vi "Main.vi"() -> ()   [LabVIEW 2021]
uses:
  <vilib>/Analysis/NI_AALBase.lvlib
  <vilib>/Analysis/Matrix/NI_Matrix.lvlib
  <vilib>/Analysis/baseanly.llb/Real Inverse Matrix.vi
  <vilib>/Analysis/Matrix/Numeric/Multiply/Multiply - RM,RM.vi
  <vilib>/Analysis/NI_AALPro.lvlib
  <vilib>/gmath/NI_Gmath.lvlib
  <vilib>/Analysis/7linalg.llb/Eigenvalue and Vectors Output Option.ctl
  <vilib>/Analysis/7linalg.llb/Real Eigenvalues and Vectors.vi
  <vilib>/Analysis/baseanly.llb/Matrix Type of Inverse Matrix.ctl
  <vilib>/Analysis/Matrix/Numeric/Conversions/Array To Matrix - RA2.vi
  <vilib>/Analysis/4window.llb/Hanning Window (DBL).vi
  <vilib>/Analysis/5stat.llb/RMS (DBL).vi
  <vilib>/DAQmx/read.llb/DAQmx Read (Analog 1D DBL 1Chan NSamp).vi
  <vilib>/Analysis/Matrix/Numeric/Add/Add - RM,RM.vi
  <vilib>/Analysis/7linalg.llb/Real Cholesky Factorization.vi
  <vilib>/Analysis/2dsp.llb/Real FFT.vi
  <vilib>/Analysis/baseanly.llb/Mean (DBL).vi
  <vilib>/Analysis/7linalg.llb/Real Generalized Eigenvalues and Vectors.vi
  <vilib>/DAQmx/write.llb/DAQmx Write (Digital 1D Bool NChan 1Samp 1Line).vi
  <vilib>/gmath/statdist.llb/Normal Moments.vi
panel:
  out "Waveform Graph":dbl[](graph)
  out "1st Nat. Freq. (Hz) 4":waveform(dbl)[](graph) caption="1st Nat. Freq. (Hz)"
  out "1st Nat. Freq. (Hz) 3":waveform(dbl)(graph) caption="Est. 1st Nat. Freq. (Hz)"
  out "Std. Dev.":dbl
  in  "error in 2":errorcluster caption="error in"
  out "time_acceleration_data":dbl[](array[numeric])
  out "XY Graph 2":cluster{dbl[], dbl[]}[](graph)
  in  "MASTER":bool
  out "XY Graph":cluster{dbl[], dbl[]}[](graph)
  out "1st Nat. Freq. (Hz)":waveform(dbl)(graph) caption="measured 1st Nat. Freq. (Hz)"
  out "Estimated Pin Node":i32[](graph)
  in  "Tab Control":T1(tab)
  in  "Frequency Method":enum16{"0-Tone", "1-FFT-CPU"}(ring)=enum."1-FFT-CPU"
  in  "Width":dbl=0.0508 format="%#.6f"
  in  "Density":dbl=7900.0
  in  "Height":dbl=0.00635
  in  "Length of Beam":dbl=0.3525
  in  "Young's Modulus":dbl=209500000000.0
  in  "Torsion Spring":dbl format="%#.6f"
  in  "Initial Pin node":i32
  in  "Std. Dev.":dbl=1.0 min=0.0
  in  "Eigenvalue Method":T2(ring)=enum."2-LabVIEW Cholesky Factorization"
  out "average cycle time (ms)":dbl format="%0.2f"
  in  "FFT data length (data points)":i32=5000
  in  "Min. FFT Power Value (RMS)":dbl=0.02
  in  "Bound to 1st Frequency":bool=TRUE
  out "Low-Energy Warning":bool
  in  "accelerometer_mass":dbl=0.055
  in  "Std. Dev = Number of Particles / 3":bool=TRUE
  out "Std. Dev.  2":dbl
  in  "Number Of Particles":i32=3
  in  "FEA Nodes":i32=40
  in  "file name":i32
  out "FFT_data_length":i32=5000
  in  "Auto FFT length":bool
  out "Hz / per pin location":dbl
  out "FFT_frequency_resolution":dbl
  in  "scaling_factor_Hz_per_pin_to_frequency_resolution":dbl=0.33 format="%#_13g"
  in  "save acceleration_data":bool=TRUE
  out "1st Nat. Freq. (Hz) 2":dbl format="%#_5g"
  out "FEA Frequencies":dbl[](array[numeric])
  out "Acceleration Data":dbl[](graph) caption="All Data"
  out "Sampled Acceleration Data":dbl[](graph) caption="Sampled Data"
  in  "Real-Time plotting":bool
  out "Probability Density Function":cluster{i32[], dbl[]}(graph)
  # "Note: All Inputs are based on base SI units."
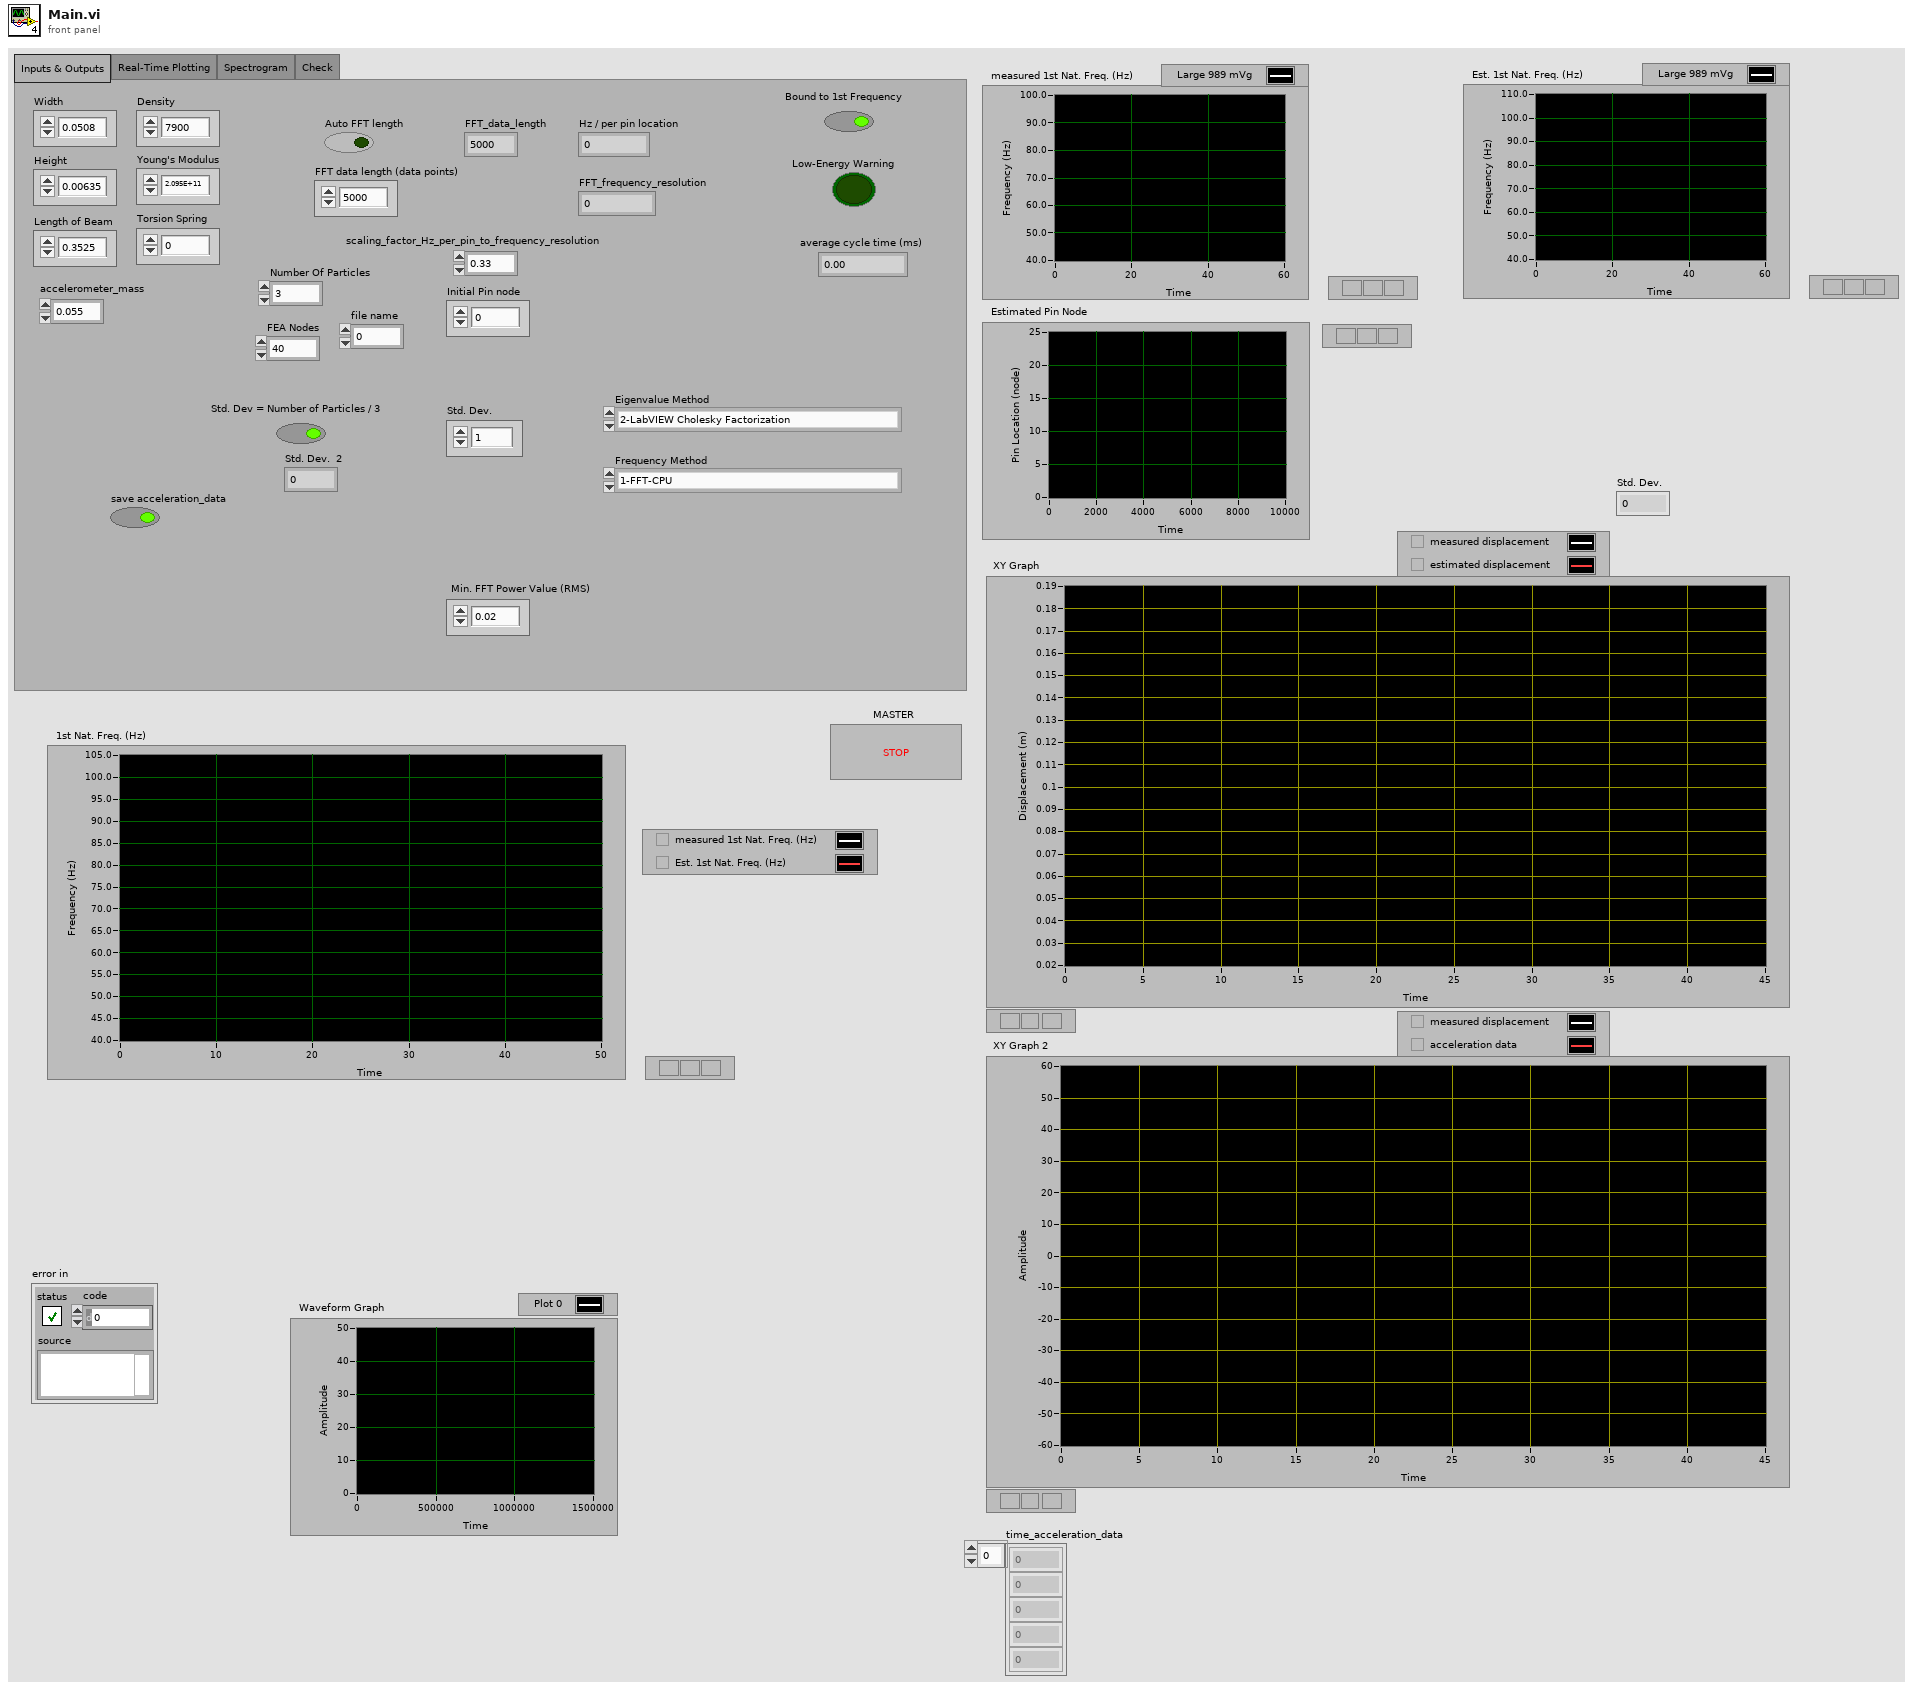
[diagram p1: front panel]
types:
  T1 = enum32{"Inputs & Outputs", "Real-Time Plotting", "Spectrogram", "Check"}
  T2 = enum16{"0-LabVIEW generalized eigenvalues", "1-LabVIEW M^-1K eigenvalues", "2-LabVIEW Cholesky Factorization", "3-Cholesky Factorization CPU SGL", "4-Cholesky Factorization CPU FXP", "5-Cholesky Factorization FPGA SGL", "6-Cholesky Factorization FPGA SGL SCL"}
  T3 = cluster{"beam_length":dbl, "youngs_modulus":dbl, "torsion_spring":dbl, "beam_height":dbl, "beam_width":dbl, "beam_density":dbl, "number_of_FEA_nodes":i32, "FFT_data_length":i32, "standard_deviation":dbl, "number_of_particles":i32, "min_FFT_power_value":dbl, "initial_pin_node":i32, "accelerometer_mass":dbl}
  T4 = cluster{"time_average_cycle":dbl, "measured_frequency":dbl[], "date_time":string, "estimated_pin_node":i32[], "time_cycle_start":dbl[], "measured_pin_location":dbl[], "estimated_frequency":dbl[], "acceleration_data":dbl[], "accelerometer_sample_rate":dbl, "displacement_sample_rate":dbl, "time_compare_start":dbl[], "time_subsample_start":dbl[], "time_FEA_start":dbl[], "time_FEA_end":dbl[], "time_cycle_end":dbl[], "time_accelerometer_aquire_start":dbl[], "time_frequency_calculations_start":dbl[], "time_frequency_calculations_end":dbl[], "measured_pin_location_tt":dbl[], "time_ACC_data_collection_start":dbl, "time_acceleration_data":dbl[], "estimated_pin_location":dbl[], "scaling_factor_Hz_per_pin_to_frequency_resolution":dbl, "Std_Dev_equale_particles_divided_3":bool, "Auto_FFT_length":bool, "windowed_acc_data":dbl[][], "FFT":dbl[][]}
  T5 = typedef "NI_AALBase.lvlib/Matrix Type of Inverse Matrix.ctl" = enum32{"General", "Positive Definite", "Lower Triangular", "Upper Triangular"}
  T6 = typedef "NI_AALPro.lvlib/Eigenvalue and Vectors Output Option.ctl" = i32
  T7 = typedef "NI_Matrix.lvlib/RealMatrix.ctl" = dbl[][]
  T8 = cluster{"measured_pin_location_tt":dbl[], "measured_pin_location":dbl[]}
  T9 = cluster{"time_acceleration_data":dbl[], "acceleration_data":dbl[]}
  T10 = cluster{"time_cycle_end":dbl[], "estimated_pin_location":dbl[]}
  T11 = cluster{"time_acceleration_data":dbl[], "acceleration_data":dbl[]}[]
  T12 = cluster{"time_cycle_end":dbl[], "estimated_pin_location":dbl[]}[]
  T13 = cluster{"time_average_cycle":dbl, "measured_frequency":dbl[], "date_time":string, "estimated_pin_node":i32[], "time_cycle_start":dbl[], "measured_pin_location":dbl[], "estimated_frequency":dbl[], "acceleration_data":dbl[], "accelerometer_sample_rate":dbl, "displacement_sample_rate":dbl, "time_compare_start":dbl[], "time_subsample_start":dbl[], "time_FEA_start":dbl[], "time_FEA_end":dbl[], "time_cycle_end":dbl[], "time_accelerometer_aquire_start":dbl[], "time_frequency_calculations_start":dbl[], "time_frequency_calculations_end":dbl[], "measured_pin_location_tt":dbl[], "time_ACC_data_collection_start":dbl, "time_acceleration_data":dbl[], "estimated_pin_location":dbl[], "scaling_factor_Hz_per_pin_to_frequency_resolution":dbl, "Std_Dev_equale_particles_divided_3":bool, "Auto_FFT_length":bool, "windowed_acc_data":dbl[][], "FFT":dbl[][], "beam_length":dbl, "youngs_modulus":dbl, "torsion_spring":dbl, "beam_height":dbl, "beam_width":dbl, "beam_density":dbl, "number_of_FEA_nodes":i32, "FFT_data_length":i32, "standard_deviation":dbl, "number_of_particles":i32, "min_FFT_power_value":dbl, "initial_pin_node":i32, "accelerometer_mass":dbl}
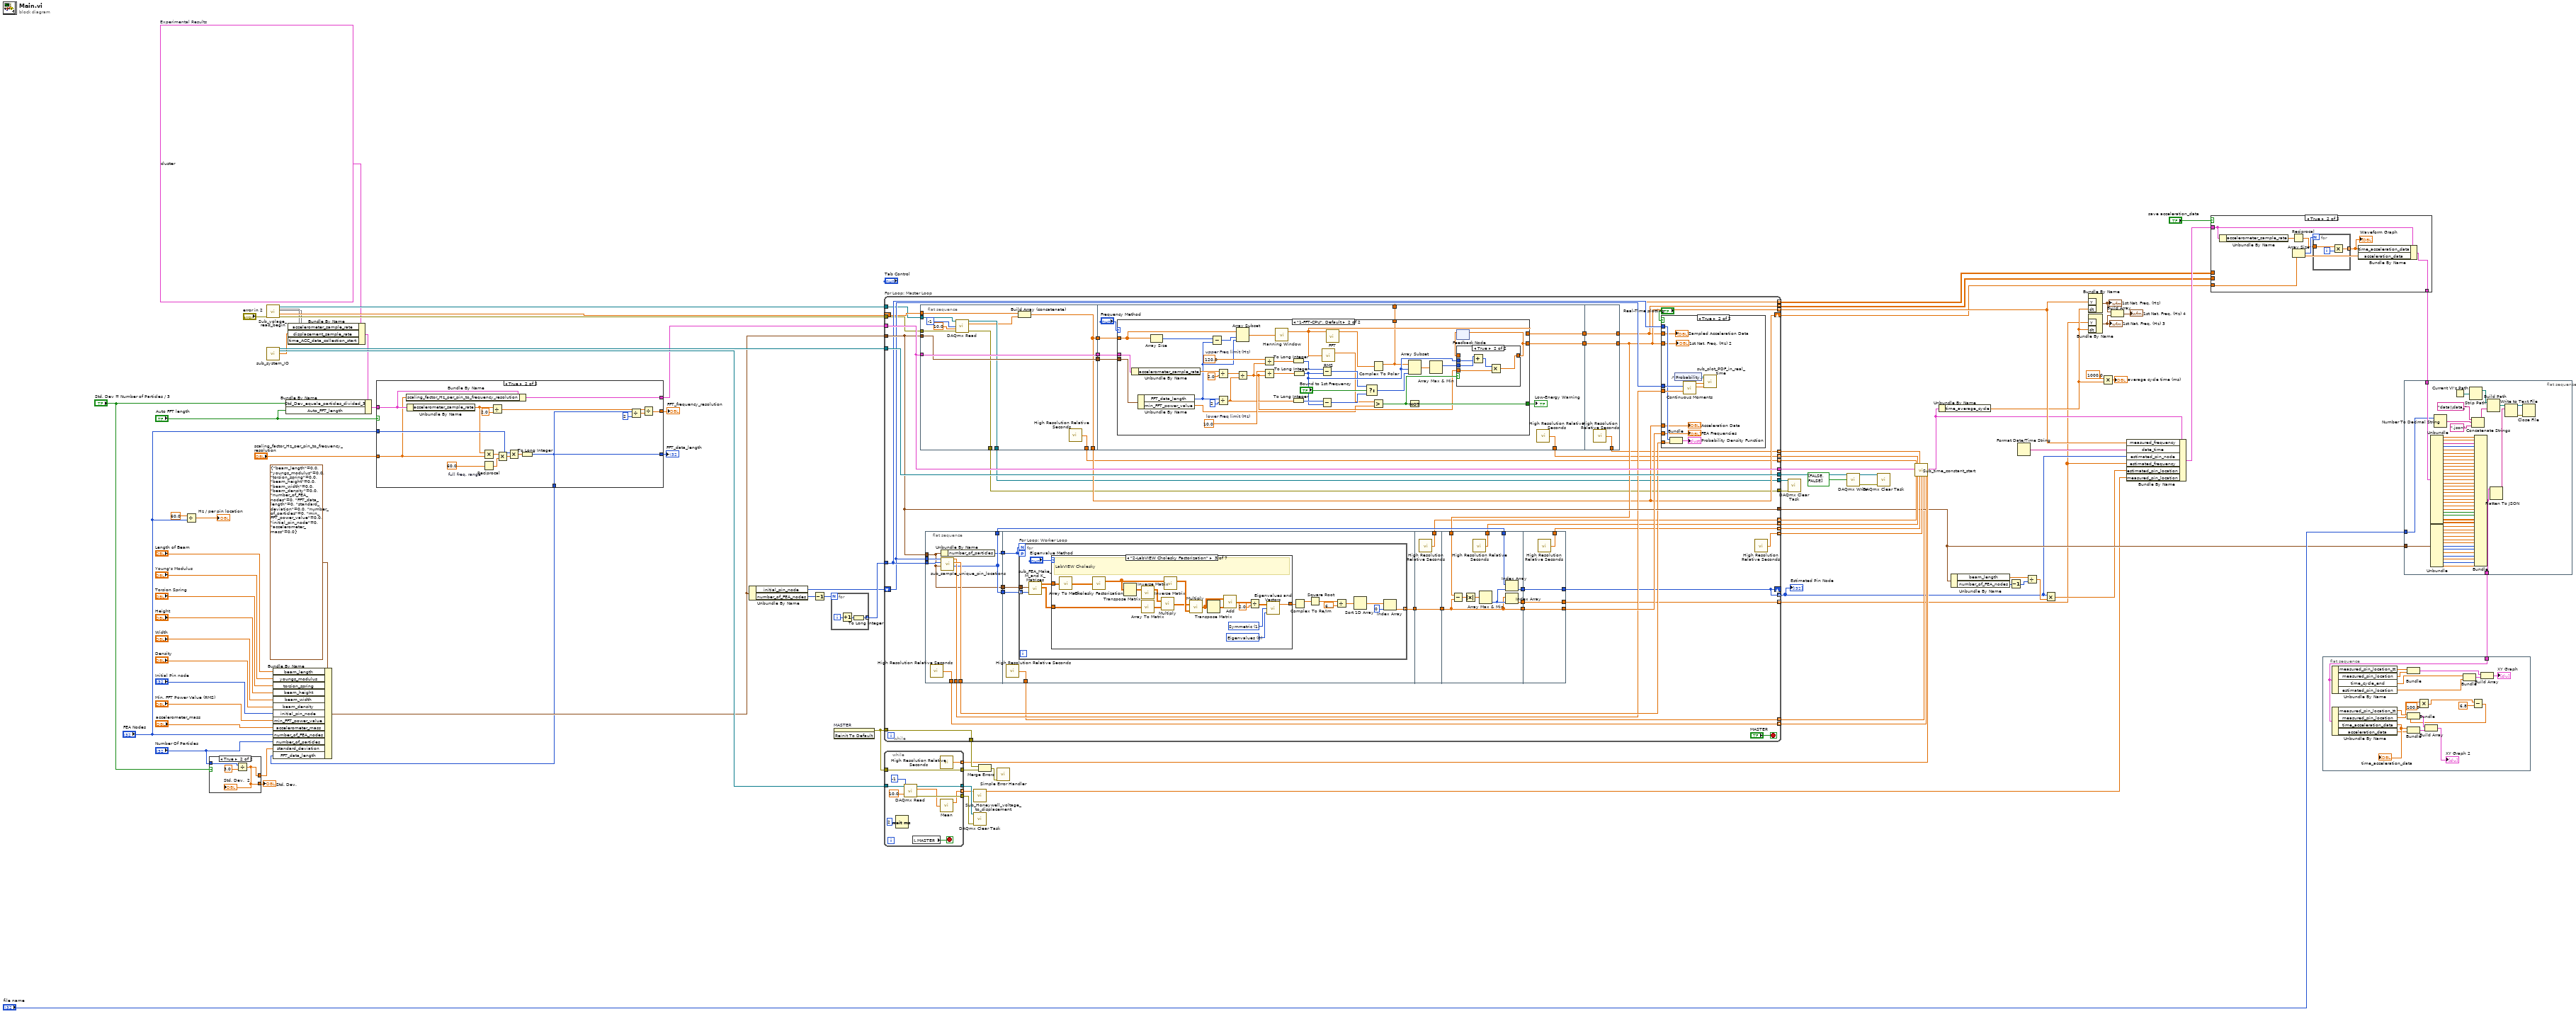
[diagram p0: block diagram]
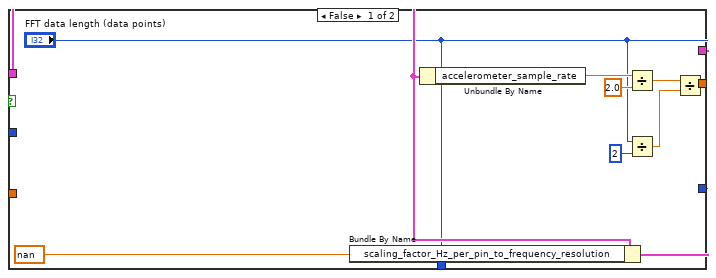
[diagram p3: hidden frame]
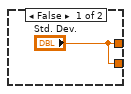
[diagram p4: hidden frame]
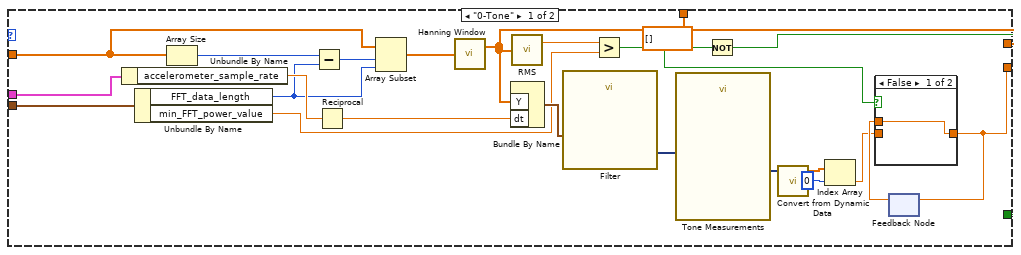
[diagram p5: hidden frame]
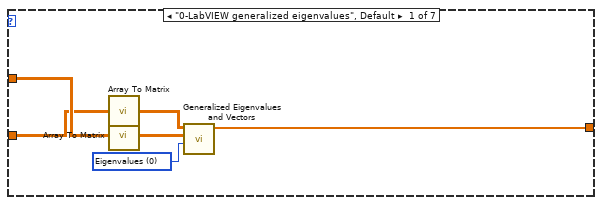
[diagram p8: hidden frame]
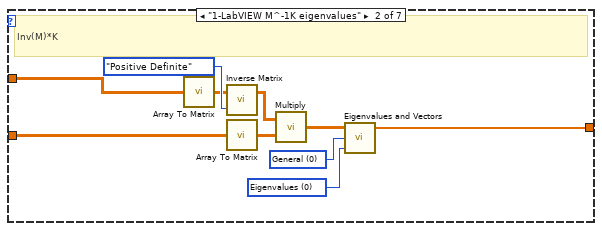
[diagram p9: hidden frame]
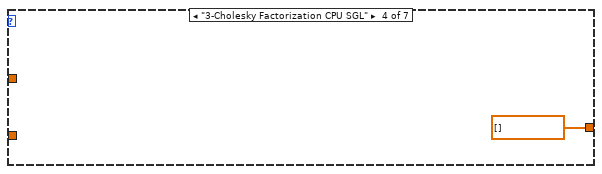
[diagram p10: hidden frame]
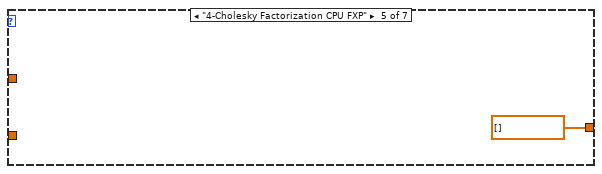
[diagram p11: hidden frame]
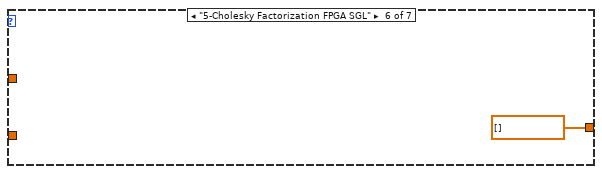
[diagram p12: hidden frame]
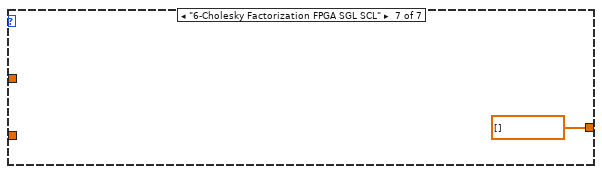
[diagram p13: hidden frame]
diagram:
  w35 = T4 {"time_average_cycle"=0.0, "measured_frequency"=[], "date_time"="", "estimated_pin_node"=[], "time_cycle_start"=[], "measured_pin_location"=[], "estimated_frequency"=[], "acceleration_data"=[], "accelerometer_sample_rate"=0.0, "displacement_sample_rate"=0.0, "time_compare_start"=array[564 elements], "time_subsample_start"=array[564 elements], "time_FEA_start"=array[564 elements], "time_FEA_end"=array[564 elements], "time_cycle_end"=array[564 elements], "time_accelerometer_aquire_start"=array[564 elements], "time_frequency_calculations_start"=array[564 elements], "time_frequency_calculations_end"=array[564 elements], "measured_pin_location_tt"=array[564 elements], "time_ACC_data_collection_start"=0.0, "time_acceleration_data"=array[564 elements], "estimated_pin_location"=array[564 elements], "scaling_factor_Hz_per_pin_to_frequency_resolution"=1.0, "Std_Dev_equale_particles_divided_3"=TRUE, "Auto_FFT_length"=TRUE, "windowed_acc_data"=array1x564[564 elements], "FFT"=array1x564[564 elements]}  # Experimental Results
  n1 = Divide(x=60.0, y="FEA Nodes") -> (x/y=→"Hz / per pin location":dbl)
  n2 = case shown="True" "Std. Dev = Number of Particles / 3" {
    tunnel: ["Std. Dev." w92] -> w12
    tunnel: "Number Of Particles" -> [_ w93]
    tunnel: ["Std. Dev." w92] -> w90
    frame False {
    }
    frame True {
      n3 = Divide(x=w93, y=3.0) -> (x/y=w92:dbl)
      "Std. Dev.  2" <- w92
    }
  }
  "Std. Dev." <- w90
  n4 = call "Sub_volage_read_begin.vi"(8:"error in 2") -> ("error out"=w47:errorcluster, "data"=w46:dbl[], 2:w44, "Task out"=w48:refnum<k21>, 5:w45)  [unwired: 5 in, 1 out]
  n5 = call "sub_system_IO.vi"() -> ("displacement task"=w71:refnum<k21>, "Parker task"=w61:refnum<k21>, "displacement sample rate (S/s)"=w15:dbl)  [unwired: 6 in, 7 out]
  n6 = Bundle By Name(cluster=w35, "accelerometer_sample_rate"=w45, "displacement_sample_rate"=w15, "time_ACC_data_collection_start"=w44) -> (w28:T4)
  n7 = Bundle By Name(cluster=w28, "Std_Dev_equale_particles_divided_3"="Std. Dev = Number of Particles / 3", "Auto_FFT_length"="Auto FFT length") -> (w25:T4)
  n8 = case shown="True" "Auto FFT length" {
    tunnel: "FEA Nodes" -> [_ w112]
    tunnel: w25 -> [w98 w109]
    tunnel: ["FFT data length (data points)" w107] -> w13
    tunnel: [w99 w111] -> w33
    tunnel: ["FFT data length (data points)" w107] -> w32
    tunnel: [w97 w108] -> w29
    tunnel: "scaling_factor_Hz_per_pin_to_frequency_resolution" -> [_ w106]
    frame False {
      n9 = Bundle By Name(cluster=w98, "scaling_factor_Hz_per_pin_to_frequency_resolution"=nan) -> (w97:T4)
      n10 = Unbundle By Name(w98) -> ("accelerometer_sample_rate"=w104:dbl)
      n11 = Divide(x=w104, y=2.0) -> (x/y=w102:dbl)
      n12 = Divide(x="FFT data length (data points)", y=2) -> (x/y=w103:dbl)
      n13 = Divide(x=w102, y=w103) -> (x/y=w99:dbl)
    }
    frame True {
      w115 = 60.0  # full freq. range
      n14 = Bundle By Name(cluster=w109, "scaling_factor_Hz_per_pin_to_frequency_resolution"=w106) -> (w108:T4)
      n15 = Unbundle By Name(w109) -> ("accelerometer_sample_rate"=w105:dbl)
      n16 = Multiply(x=w105, y=w106) -> (x*y=w118:dbl)
      n17 = Reciprocal(x=w115) -> (1/x=w119:dbl)
      n18 = Divide(x=w105, y=2.0) -> (x/y=w116:dbl)
      n19 = Multiply(x=w118, y=w119) -> (x*y=w120:dbl)
      n20 = Multiply(x=w112, y=w120) -> (x*y=w110:dbl)
      n21 = To Long Integer(number=w110) -> (32bit integer=w107:i32)
      n22 = Divide(x=w107, y=2) -> (x/y=w117:dbl)
      n23 = Divide(x=w116, y=w117) -> (x/y=w111:dbl)
    }
  }
  "FFT_frequency_resolution" <- w33
  "FFT_data_length" <- w32
  n24 = Bundle By Name(cluster=T3 {"beam_length"=0.0, "youngs_modulus"=0.0, "torsion_spring"=0.0, "beam_height"=0.0, "beam_width"=0.0, "beam_density"=0.0, "number_of_FEA_nodes"=0, "FFT_data_length"=0, "standard_deviation"=0.0, "number_of_particles"=0, "min_FFT_power_value"=0.0, "initial_pin_node"=0, "accelerometer_mass"=0.0} ("Setup Parameters"), "beam_length"="Length of Beam", "youngs_modulus"="Young's Modulus", "torsion_spring"="Torsion Spring", "beam_height"="Height", "beam_width"="Width", "beam_density"="Density", "initial_pin_node"="Initial Pin node", "min_FFT_power_value"="Min. FFT Power Value (RMS)", "accelerometer_mass"="accelerometer_mass", "number_of_FEA_nodes"="FEA Nodes", "number_of_particles"="Number Of Particles", "standard_deviation"=w12, "FFT_data_length"=w13) -> (w34:T3)
  n25 = Unbundle By Name(w34) -> ("initial_pin_node"=w64:i32, "number_of_FEA_nodes"=w59:i32)
  n26 = Decrement(x=w59) -> (x-1=w88:i32)
  n27 = for {
    N: w88 -> [_]
    tunnel: [w123] -> w89 mode=indexing
    i -> [w121]
    n28 = Increment(x=w121) -> (x+1=w122:i32)
    n29 = To Long Integer(number=w122) -> (32bit integer=w123:i32)
  }
  n30 = invoke on="MASTER" class="Bool (strict)" method="Reinit To Default"() -> (error out=w68:errorcluster)  [unwired: 3 in, 2 out]
  n31 = while "For Loop: Master Loop" {
    shift-right: [w153] -> _
    shift-left: w64 -> [w156]
    tunnel: [w152] -> w3 mode=indexing
    tunnel: w89 -> [w157]
    tunnel: [w153] -> w6 mode=indexing
    tunnel: w48 -> [w146]
    tunnel: [w143] -> w86
    tunnel: [w144] -> w85
    shift-right: [w147] -> w21
    shift-left: w46 -> [w148]
    tunnel: w61 -> [w166]
    tunnel: [w166] -> w81
    tunnel: [w154] -> w73 mode=indexing
    tunnel: w34 -> [w163]
    tunnel: [w165] -> w66
    tunnel: w68 -> [w165]
    tunnel: w29 -> [w164]
    tunnel: [w164] -> w42
    tunnel: [w163] -> w40
    tunnel: w47 -> [w145]
    tunnel: [w137] -> w53 mode=indexing
    tunnel: [w136] -> w7 mode=indexing
    tunnel: [w135] -> w56 mode=indexing
    tunnel: [w134] -> w51 mode=indexing
    tunnel: [w133] -> w54 mode=indexing
    tunnel: [w132] -> w55 mode=indexing
    tunnel: [w126] -> w57 mode=indexing
    tunnel: [w129] -> w50 mode=indexing
    tunnel: [w128] -> w52 mode=indexing
    tunnel: [w125] -> w2 mode=indexing
    tunnel: [w124] -> w1 mode=indexing
    stop <- "MASTER" stop-if-true
    n32 = flat-sequence {
      tunnel: w163 -> [w179]
      tunnel: w164 -> [w180]
      tunnel: [w180] -> w151
      tunnel: [w177] -> w150
      tunnel: [w179] -> w149
      tunnel: w148 -> [w178]
      tunnel: [w177] -> w147
      tunnel: w146 -> [w174]
      tunnel: w145 -> [w173]
      tunnel: [w172] -> w144
      tunnel: [w171] -> w143
      tunnel: [w169] -> w134
      tunnel: w151 -> [w187]
      tunnel: w150 -> [w186]
      tunnel: w149 -> [w185]
      tunnel: [w189] -> w139
      tunnel: [w184] -> w138
      tunnel: [w182] -> w133
      tunnel: [w181] -> w124
      tunnel: [w257] -> w154
      tunnel: [w258] -> w125
      tunnel: w139 -> [w258]
      tunnel: w138 -> [w257]
      tunnel: [w256] -> w132
      frame #0 {
        n33 = call-poly <vilib>:"DAQmx Read.vi"("task/channels in"=w174, "number of samples per channel"=-1 ("number of samples"), "timeout"=10.0 ("timeout (s)"), "error in"=w173) -> ("task out"=w171:refnum<k21>, "data"=w170:dbl[], "error out"=w172:errorcluster)  [unwired: 9 in]
        n34 = Build Array (concatenate)(w178, w170) -> (w177:dbl[])
        n35 = call <vilib>:"High Resolution Relative Seconds.vi"() -> ("relative seconds"=w169:dbl)
      }
      frame #1 {
        n36 = case shown="\"1-FFT-CPU\", Default" "Frequency Method" {
          tunnel: [w200 w236] -> w184
          tunnel: [w202 w216] -> w189
          tunnel: w186 -> [w204 w238]
          tunnel: [w197 w232] -> w188
          tunnel: w185 -> [w193 w221]
          tunnel: w187 -> [w195 w219]
          tunnel: [dbl[] [] w215] -> w181
          frame "0-Tone" {
            n37 = Unbundle By Name(w195) -> ("accelerometer_sample_rate"=w194:dbl)
            n38 = Unbundle By Name(w193) -> ("FFT_data_length"=w191:i32, "min_FFT_power_value"=w192:dbl)
            n39 = Array Size(array=w204) -> (size(s)=w212:i32)
            n40 = Subtract(x=w212, y=w191) -> (x-y=w211:i32)
            n41 = Reciprocal(x=w194) -> (1/x=w196:dbl)
            n42 = Array Subset(array=w204, index=w211, length=w191) -> (w205:dbl[])
            n43 = call-poly <vilib>:"Hanning Window.vi"("X"=w205) -> ("Windowed X"=w202:dbl[])  [unwired: 1 out]
            n44 = Bundle By Name("Y"=w202, "dt"=w196) -> (w206:waveform(dbl))  [unwired: 1 in]
            n45 = call-poly <vilib>:"RMS.vi"("X"=w202) -> ("rms value"=w198:dbl)  [unwired: 1 out]
            n46 = call "Filter"("Signal"=w206) -> ("Filtered Signal"=w207:dynamicdata)  [unwired: 9 in, 1 out]
            n47 = Greater?(x=w198, y=w192) -> (0:w199:bool)
            n48 = call "Tone Measurements"("Signals"=w207) -> ("Frequency"=w208:dynamicdata)  [unwired: 9 in, 1 out]
            n49 = Not(x=w199) -> (.not. x?=w197:bool)
            n50 = call "Convert from Dynamic Data"("Dynamic Data Type"=w208) -> ("Array"=w209:dbl[])  [unwired: 3 in]
            n51 = Index Array(array=w209, index=0) -> (element=w201:dbl)
            n52 = feedback #1() -> (w203:dbl)  [unwired: 1 in]
            n53 = case shown="False" w199 {
              tunnel: [w213 w214] -> w200
              tunnel: w203 -> [w213 _]
              tunnel: w201 -> [_ w214]
              frame False {
              }
              frame True {
              }
            }
            n54 = feedback-in #1(w200) -> ()
          }
          frame "1-FFT-CPU", Default {
            w231 = 120.0  # upper Freq limit (Hz)
            w248 = 10.0  # lower Freq limit (Hz)
            n55 = Unbundle By Name(w219) -> ("accelerometer_sample_rate"=w218:dbl)
            n56 = Unbundle By Name(w221) -> ("FFT_data_length"=w217:i32, "min_FFT_power_value"=w220:dbl)
            n57 = Array Size(array=w238) -> (size(s)=w240:i32)
            n58 = Subtract(x=w240, y=w217) -> (x-y=w239:i32)
            n59 = Divide(x=w218, y=2.0) -> (x/y=w242:dbl)
            n60 = Divide(x=w217, y=2) -> (x/y=w241:dbl)
            n61 = Array Subset(array=w238, index=w239, length=w217) -> (w237:dbl[])
            n62 = Divide(x=w242, y=w241) -> (x/y=w230:dbl)
            n63 = Divide(x=w231, y=w230) -> (x/y=w229:dbl)
            n64 = Divide(x=w248, y=w230) -> (x/y=w247:dbl)
            n65 = call-poly <vilib>:"Hanning Window.vi"("X"=w237) -> ("Windowed X"=w216:dbl[])  [unwired: 1 out]
            n66 = To Long Integer(number=w229) -> (32bit integer=w228:i32)
            n67 = To Long Integer(number=w241) -> (32bit integer=w244:i32)
            n68 = To Long Integer(number=w247) -> (32bit integer=w227:i32)
            n69 = Subtract(x=w228, y=w227) -> (x-y=w224:i32)
            n70 = Subtract(x=w244, y=w227) -> (x-y=w223:i32)
            n71 = call-poly <vilib>:"RMS.vi"("X"=w216) -> ("rms value"=w222:dbl)  [unwired: 1 out]
            n72 = call-poly <vilib>:"FFT.vi"("X"=w216) -> ("FFT {X}"=w245:cdb[])  [unwired: 9 in, 1 out]
            n73 = Select(t=w224, s="Bound to 1st Frequency", f=w223) -> (s? t:f=w226:i32)
            n74 = Greater?(x=w222, y=w220) -> (0:w233:bool)
            n75 = Complex To Polar(r * e^(i*theta)=w245) -> (r=w215:dbl[])  [unwired: 1 out]
            n76 = Not(x=w233) -> (.not. x?=w232:bool)
            n77 = Array Subset(array=w215, index=w227, length=w226) -> (w234:dbl[])
            n78 = Array Max & Min(array=w234) -> (max index (indices)=w246:i32)  [unwired: 3 out]
            n79 = feedback #2() -> (w235:dbl)  [unwired: 1 in]
            n80 = case shown="True" w233 {
              tunnel: w246 -> [_ w255]
              tunnel: w227 -> [_ w253]
              tunnel: w230 -> [_ w252]
              tunnel: [w250 w251] -> w236
              tunnel: w235 -> [w250 _]
              frame False {
              }
              frame True {
                n81 = Add(x=w255, y=w253) -> (x+y=w254:i32)
                n82 = Multiply(x=w254, y=w252) -> (x*y=w251:dbl)
              }
            }
            n83 = feedback-in #2(w236) -> ()
          }
        }
        "Low-Energy Warning" <- w188
        n84 = call <vilib>:"High Resolution Relative Seconds.vi"() -> ("relative seconds"=w182:dbl)
      }
      frame #2 {
        n85 = call <vilib>:"High Resolution Relative Seconds.vi"() -> ("relative seconds"=w256:dbl)
      }
    }
    n86 = flat-sequence {
      tunnel: w163 -> [w259]
      tunnel: [w262] -> w162
      tunnel: [w259] -> w161
      tunnel: [w261] -> w160
      tunnel: [w266] -> w159
      tunnel: [w265] -> w158
      tunnel: w157 -> [w264]
      tunnel: w156 -> [w263]
      tunnel: [w262] -> w155
      tunnel: [w260] -> w137
      tunnel: w162 -> [w271]
      tunnel: w161 -> [w269]
      tunnel: w160 -> [w267]
      tunnel: [w270] -> w131
      tunnel: [w268] -> w136
      tunnel: w131 -> [w323]
      tunnel: [w323] -> w130
      tunnel: [w322] -> w129
      tunnel: w130 -> [w328]
      tunnel: w155 -> [w329]
      tunnel: w154 -> [w327]
      tunnel: [w328] -> w142
      tunnel: [w326] -> w141
      tunnel: [w325] -> w140
      tunnel: [w324] -> w135
      tunnel: [w334] -> w152
      tunnel: [w335] -> w153
      tunnel: [w336] -> w167
      tunnel: w142 -> [w336]
      tunnel: w141 -> [w335]
      tunnel: w140 -> [w334]
      tunnel: [w333] -> w128
      frame #0 {
        n87 = call <vilib>:"High Resolution Relative Seconds.vi"() -> ("relative seconds"=w260:dbl)
        n88 = Unbundle By Name(w259) -> ("number_of_particles"=w261:i32)
        n89 = call "sub_sample_unique_pin_locations.vi"("Setup Parameters"=w259, "FEA Nodes"=w264, "Initial Pin Location"=w263) -> ("Unique Samples"=w262:i32[], "Sample PDF"=w266:dbl[], "Standard Deviation"=w265:dbl)  [unwired: 6 in]
      }
      frame #1 {
        n90 = call <vilib>:"High Resolution Relative Seconds.vi"() -> ("relative seconds"=w268:dbl)
        n91 = for "For Loop: Worker Loop" {
          N: w267 -> [_]
          tunnel: [w279] -> w270 mode=indexing
          tunnel: w271 -> [w276] mode=indexing
          tunnel: w269 -> [w272]
          workers-P: w267 -> [_]
          n92 = call "sub_FEA_Make_M_and K_Matrices.vi"("Pin Location"=w276, 10:w272) -> ("K Matrix"=w275:dbl[][], "M Matrix"=w274:dbl[][])  [unwired: 8 in]
          n93 = case shown="\"2-LabVIEW Cholesky Factorization\"" "Eigenvalue Method" {
            tunnel: w274 -> [w288 w294 w302 _ _ _ _]
            tunnel: w275 -> [w287 w292 w304 _ _ _ _]
            tunnel: [w289 w297 w305 cdb[] [] ("Eigenvalues") cdb[] [] ("Eigenvalues") cdb[] [] ("Eigenvalues") cdb[] [] ("Eigenvalues")] -> w277
            frame "0-LabVIEW generalized eigenvalues", Default {
              w290 = T6 0 items=["Eigenvalues", "Eigenvalues & Vectors"] ("output option")
              n94 = call-poly <vilib>:"Array To Matrix.vi"("Real 2D Array"=w287) -> ("Real Matrix"=w286:T7)
              n95 = call-poly <vilib>:"Array To Matrix.vi"("Real 2D Array"=w288) -> ("Real Matrix"=w285:T7)
              n96 = call-poly <vilib>:"Generalized Eigenvalues and Vectors.vi"("output option"=w290, "B"=w285, "A"=w286) -> ("Eigenvalues"=w289:cdb[])  [unwired: 3 in, 2 out]
            }
            frame "1-LabVIEW M^-1K eigenvalues" {
              w296 = T6 0 items=["Eigenvalues", "Eigenvalues & Vectors"] ("output option")
              w299 = 0 items=["General", "Symmetric"] ("matrix type")
              # "Inv(M)*K"
              n97 = call-poly <vilib>:"Array To Matrix.vi"("Real 2D Array"=w294) -> ("Real Matrix"=w293:T7)
              n98 = call-poly <vilib>:"Inverse Matrix.vi"("matrix type"=Matrix_Type_of_Inverse_Matrix."Positive Definite", "Input Matrix"=w293) -> ("Inverse Matrix"=w300:T7)  [unwired: 1 out]
              n99 = call-poly <vilib>:"Array To Matrix.vi"("Real 2D Array"=w292) -> ("Real Matrix"=w291:T7)
              n100 = call-poly <vilib>:"Multiply.vi"("Real Matrix B"=w291, "Real Matrix A"=w300) -> ("A * B"=w298:T7)
              n101 = call-poly <vilib>:"Eigenvalues and Vectors.vi"("output option"=w296, "matrix type"=w299, "Input Matrix"=w298) -> ("Eigenvalues"=w297:cdb[])  [unwired: 2 out]
            }
            frame "2-LabVIEW Cholesky Factorization" {
              w307 = T6 0 items=["Eigenvalues", "Eigenvalues & Vectors"] ("output option")
              w308 = 1 items=["General", "Symmetric"] ("matrix type")
              # "LabVIEW Cholesky"
              n102 = call-poly <vilib>:"Array To Matrix.vi"("Real 2D Array"=w302) -> ("Real Matrix"=w301:T7)
              n103 = call-poly <vilib>:"Cholesky Factorization.vi"("A"=w301) -> ("Cholesky"=w316:T7)  [unwired: 1 out]
              n104 = Transpose Matrix(1:w316) -> (0:w317:T7)
              n105 = call-poly <vilib>:"Inverse Matrix.vi"("Input Matrix"=w317) -> ("Inverse Matrix"=w315:T7)  [unwired: 1 in, 1 out]
              n106 = call-poly <vilib>:"Array To Matrix.vi"("Real 2D Array"=w304) -> ("Real Matrix"=w303:T7)
              n107 = call-poly <vilib>:"Multiply.vi"("Real Matrix B"=w303, "Real Matrix A"=w315) -> ("A * B"=w313:T7)
              n108 = call-poly <vilib>:"Inverse Matrix.vi"("Input Matrix"=w316) -> ("Inverse Matrix"=w314:T7)  [unwired: 1 in, 1 out]
              n109 = call-poly <vilib>:"Multiply.vi"("Real Matrix B"=w314, "Real Matrix A"=w313) -> ("A * B"=w312:T7)
              n110 = Transpose Matrix(1:w312) -> (0:w311:T7)
              n111 = call-poly <vilib>:"Add.vi"("Real Matrix B"=w311, "Real Matrix A"=w312) -> ("A + B"=w309:T7)
              n112 = Divide(x=w309, y=2.0) -> (x/y=w306:T7)
              n113 = call-poly <vilib>:"Eigenvalues and Vectors.vi"("output option"=w307, "matrix type"=w308, "Input Matrix"=w306) -> ("Eigenvalues"=w305:cdb[])  [unwired: 2 out]
            }
            frame "3-Cholesky Factorization CPU SGL" {
            }
            frame "4-Cholesky Factorization CPU FXP" {
            }
            frame "5-Cholesky Factorization FPGA SGL" {
            }
            frame "6-Cholesky Factorization FPGA SGL SCL" {
            }
          }
          n114 = Complex To Re/Im ("Complex To Cartesian.vi")(x + iy=w277) -> (x=w284:dbl[])  [unwired: 1 out]
          n115 = Square Root ("Square Root.vi")(x=w284) -> (sqrt(x)=w283:dbl[])
          n116 = Divide(x=w283, y=6.283185307179586) -> (x/y=w278:dbl[])
          n117 = Sort 1D Array(array=w278) -> (sorted array=w281:dbl[])
          n118 = Index Array(array=w281, index=0) -> (element=w279:dbl)
        }
      }
      frame #2 {
        n119 = call <vilib>:"High Resolution Relative Seconds.vi"() -> ("relative seconds"=w322:dbl)
      }
      frame #3 {
        n120 = Subtract(x=w327, y=w328) -> (x-y=w332:dbl[])
        n121 = Absolute Value(x=w332) -> (abs(x)=w331:dbl[])
        n122 = call <vilib>:"High Resolution Relative Seconds.vi"() -> ("relative seconds"=w324:dbl)
        n123 = Array Max & Min(array=w331) -> (min index (indices)=w330:i32)  [unwired: 3 out]
        n124 = Index Array(array=w329, index=w330) -> (element=w326:i32)
        n125 = Index Array(array=w328, index=w330) -> (element=w325:dbl)
      }
      frame #4 {
        n126 = call <vilib>:"High Resolution Relative Seconds.vi"() -> ("relative seconds"=w333:dbl)
      }
    }
    n127 = case shown="True" "Real-Time plotting" {
      tunnel: w158 -> [_ w345]
      tunnel: w156 -> [_ w343]
      tunnel: w157 -> [_ w342]
      tunnel: w159 -> [_ w341]
      tunnel: w167 -> [_ w340]
      tunnel: w125 -> [_ w337]
      tunnel: w147 -> [_ w339]
      tunnel: w154 -> [_ w338]
      frame False {
      }
      frame True {
        n128 = Bundle(w342, "Sample PDF"=w341) -> (→"Probability Density Function":cluster{i32[], "Sample PDF":dbl[]})  [unwired: 1 in]
        n129 = control-ref of="Probability Density Function"() -> (w346:refnum<vi>)
        n130 = call-poly <vilib>:"Continuous Moments.vi"("std"=w345, "mean"=w343) -> ("variance"=w348:dbl, "mean"=w344:dbl)  [unwired: 7 in, 1 out]
        n131 = call "sub_plot_PDF_in_real_time.vi"("mean"=w344, "variance"=w348, "XYGraph in"=w346) -> ()  [unwired: 9 in]
        "FEA Frequencies" <- w340
        "Sampled Acceleration Data" <- w337
        "Acceleration Data" <- w339
        "1st Nat. Freq. (Hz) 2" <- w338
      }
    }
    n132 = call <vilib>:"High Resolution Relative Seconds.vi"() -> ("relative seconds"=w126:dbl)
  }
  "Estimated Pin Node" <- w6
  n133 = while {
    tunnel: w71 -> [w356]
    tunnel: [w351] -> w60 mode=indexing
    tunnel: [w355] -> w70
    tunnel: [w354] -> w69
    tunnel: [w359] -> w67
    tunnel: w68 -> [w359]
    tunnel: [w353] -> w58 mode=indexing
    stop <- w358 stop-if-true
    n134 = Wait (ms)(milliseconds to wait=u32 2) -> ()  [unwired: 1 out]
    n135 = call-poly <vilib>:"DAQmx Read.vi"("task/channels in"=w356, "number of samples per channel"=-1, "timeout"=10.0 ("timeout (s)")) -> ("task out"=w355:refnum<k21>, "data"=w349:dbl[], "error out"=w354:errorcluster)  [unwired: 10 in]
    n136 = local read "MASTER"() -> (w358:bool)
    n137 = call <vilib>:"High Resolution Relative Seconds.vi"() -> ("relative seconds"=w353:dbl)
    n138 = call-poly <vilib>:"Mean.vi"("X"=w349) -> ("mean"=w351:dbl)  [unwired: 1 out]
  }
  n139 = call "Sub_Honeywell_voltage_to_displacement.vi"("Pin location voltage"=w60) -> ("Pin location meters"=w5:dbl[])  [unwired: 10 in]
  n140 = call <vilib>:"DAQmx Clear Task.vi"("task in"=w70, "error in"=w69) -> ()  [unwired: 13 in, 1 out]
  n141 = Merge Errors(w66, w67) -> (w65:errorcluster)
  n142 = call <vilib>:"Simple Error Handler.vi"("error in (no error)"=w65) -> ()  [unwired: 4 in, 5 out]
  n143 = call <vilib>:"DAQmx Clear Task.vi"("task in"=w86, "error in"=w85) -> ()  [unwired: 13 in, 1 out]
  n144 = call-poly <vilib>:"DAQmx Write.vi"("task/channels in"=w81, "data"=bool[] [FALSE, FALSE]) -> ("task out"=w83:refnum<k21>, "error out"=w82:errorcluster)  [unwired: 11 in, 1 out]
  n145 = call <vilib>:"DAQmx Clear Task.vi"("task in"=w83, "error in"=w82) -> ()  [unwired: 13 in, 1 out]
  n146 = call "Sub_time_constant_start.vi"("Array 7"=w54, "Array 3"=w51, "Experimental Results IN"=w42, "Array 6"=w53, "Array in"=w50, "Array 8"=w55, "Array 9"=w56, "Array 12"=w58, "Array 4"=w52, "Array 11"=w57, "Array 5"=w7) -> ("Experimental Results OUT"=w20:T4)  [unwired: 8 in]
  n147 = Unbundle By Name(w20) -> ("time_average_cycle"=w19:dbl)
  n148 = Unbundle By Name(w40) -> ("beam_length"=w39:dbl, "number_of_FEA_nodes"=w41:i32)
  n149 = Decrement(x=w41) -> (x-1=w38:i32)
  n150 = Format Date/Time String() -> (date/time string=w72:string)  [unwired: 3 in]
  n151 = Divide(x=w39, y=w38) -> (x/y=w37:dbl)
  n152 = Multiply(x=w6, y=w37) -> (x*y=w4:dbl[])
  n153 = Bundle By Name("Y"=w73, "dt"=w19) -> (w18:waveform(dbl))  [unwired: 1 in]
  "1st Nat. Freq. (Hz)" <- w18
  n154 = Bundle By Name("Y"=w3, "dt"=w19) -> (w17:waveform(dbl))  [unwired: 1 in]
  "1st Nat. Freq. (Hz) 3" <- w17
  n155 = Multiply(x=1000.0, y=w19) -> (x*y=→"average cycle time (ms)":dbl)
  n156 = Build Array(w18, w17) -> (→"1st Nat. Freq. (Hz) 4":waveform(dbl)[])
  n157 = Bundle By Name(cluster=w20, "measured_frequency"=w73, "date_time"=w72, "estimated_pin_node"=w6, "estimated_frequency"=w3, "estimated_pin_location"=w4, "measured_pin_location"=w5) -> (w23:T4)
  n158 = case shown="True" "save acceleration_data" {
    tunnel: [w360 w367] -> w22
    tunnel: w23 -> [w360 w366]
    tunnel: w21 -> [_ w365]
    tunnel: w2 -> [_ _]
    tunnel: w1 -> [_ _]
    frame False {
    }
    frame True {
      n159 = Unbundle By Name(w366) -> ("accelerometer_sample_rate"=w361:dbl)
      n160 = Reciprocal(x=w361) -> (1/x=w362:dbl)
      n161 = Array Size(array=w365) -> (size(s)=w363:i32)
      n162 = for {
        N: w363 -> [_]
        tunnel: w362 -> [w369]
        tunnel: [w368] -> w364 mode=indexing
        i -> [w370]
        n163 = Multiply(x=w369, y=w370) -> (x*y=w368:dbl)
      }
      "Waveform Graph" <- w364
      n164 = Bundle By Name(cluster=w366, "time_acceleration_data"=w364, "acceleration_data"=w365) -> (w367:T4)
    }
  }
  n165 = flat-sequence {
    tunnel: w36 -> [w374]
    frame #0 {
      n166 = Unbundle By Name(w374) -> ("measured_pin_location_tt"=w388:dbl[], "measured_pin_location"=w373:dbl[], "time_cycle_end"=w387:dbl[], "estimated_pin_location"=w372:dbl[])
      n167 = Unbundle By Name(w374) -> ("measured_pin_location_tt"=w386:dbl[], "measured_pin_location"=w380:dbl[], "time_acceleration_data"=w384:dbl[], "acceleration_data"=w383:dbl[])
      "time_acceleration_data" <- w384
      n168 = Bundle("measured_pin_location_tt"=w388, "measured_pin_location"=w373) -> (w389:T8)  [unwired: 1 in]
      n169 = Bundle("time_acceleration_data"=w384, "acceleration_data"=w383) -> (w381:T9)  [unwired: 1 in]
      n170 = Multiply(x=w380, y=100.0 ("x")) -> (x*y=w377:dbl[])
      n171 = Bundle("time_cycle_end"=w387, "estimated_pin_location"=w372) -> (w371:T10)  [unwired: 1 in]
      n172 = Subtract(x=w377, y=6.8) -> (x-y=w376:dbl[])
      n173 = Bundle("measured_pin_location_tt"=w386, w376) -> (w385:cluster{"measured_pin_location_tt":dbl[], dbl[]})  [unwired: 1 in]
      n174 = Build Array(w385, w381) -> (→"XY Graph 2":T11)
      n175 = Build Array(w389, w371) -> (→"XY Graph":T12)
    }
  }
  n176 = flat-sequence {
    tunnel: w40 -> [w419]
    tunnel: w22 -> [w415]
    tunnel: "file name" -> [w410]
    tunnel: [w408] -> w36
    frame #0 {
      n177 = Unbundle(w415) -> ("time_average_cycle"=w420:dbl, "measured_frequency"=w421:dbl[], "date_time"=w422:string, "estimated_pin_node"=w423:i32[], "time_cycle_start"=w424:dbl[], "measured_pin_location"=w425:dbl[], "estimated_frequency"=w426:dbl[], "acceleration_data"=w427:dbl[], "accelerometer_sample_rate"=w428:dbl, "displacement_sample_rate"=w429:dbl, "time_compare_start"=w430:dbl[], "time_subsample_start"=w431:dbl[], "time_FEA_start"=w432:dbl[], "time_FEA_end"=w433:dbl[], "time_cycle_end"=w434:dbl[], "time_accelerometer_aquire_start"=w435:dbl[], "time_frequency_calculations_start"=w436:dbl[], "time_frequency_calculations_end"=w437:dbl[], "measured_pin_location_tt"=w418:dbl[], "time_ACC_data_collection_start"=w417:dbl, "time_acceleration_data"=w416:dbl[], "estimated_pin_location"=w409:dbl[], "scaling_factor_Hz_per_pin_to_frequency_resolution"=w407:dbl, "Std_Dev_equale_particles_divided_3"=w406:bool, "Auto_FFT_length"=w405:bool, "windowed_acc_data"=w404:dbl[][], "FFT"=w403:dbl[][])
      n178 = Unbundle(w419) -> ("beam_length"=w402:dbl, "youngs_modulus"=w401:dbl, "torsion_spring"=w400:dbl, "beam_height"=w399:dbl, "beam_width"=w398:dbl, "beam_density"=w397:dbl, "number_of_FEA_nodes"=w396:i32, "FFT_data_length"=w395:i32, "standard_deviation"=w394:dbl, "number_of_particles"=w393:i32, "min_FFT_power_value"=w392:dbl, "initial_pin_node"=w391:i32, "accelerometer_mass"=w390:dbl)
      n179 = Number To Decimal String(number=w410) -> (decimal integer string=w411:string)  [unwired: 1 in]
      n180 = Current VI's Path() -> (path=w440:path)
      n181 = Strip Path(path=w440) -> (stripped path=w439:path)  [unwired: 1 out]
      n182 = Concatenate Strings("data\\data_" ("name or relative path"), w411, ".json" ("name or relative path")) -> (w412:string)
      n183 = Bundle("time_average_cycle"=w420, "measured_frequency"=w421, "date_time"=w422, "estimated_pin_node"=w423, "time_cycle_start"=w424, "measured_pin_location"=w425, "estimated_frequency"=w426, "acceleration_data"=w427, "accelerometer_sample_rate"=w428, "displacement_sample_rate"=w429, "time_compare_start"=w430, "time_subsample_start"=w431, "time_FEA_start"=w432, "time_FEA_end"=w433, "time_cycle_end"=w434, "time_accelerometer_aquire_start"=w435, "time_frequency_calculations_start"=w436, "time_frequency_calculations_end"=w437, "measured_pin_location_tt"=w418, "time_ACC_data_collection_start"=w417, "time_acceleration_data"=w416, "estimated_pin_location"=w409, "scaling_factor_Hz_per_pin_to_frequency_resolution"=w407, "Std_Dev_equale_particles_divided_3"=w406, "Auto_FFT_length"=w405, "windowed_acc_data"=w404, "FFT"=w403, "beam_length"=w402, "youngs_modulus"=w401, "torsion_spring"=w400, "beam_height"=w399, "beam_width"=w398, "beam_density"=w397, "number_of_FEA_nodes"=w396, "FFT_data_length"=w395, "standard_deviation"=w394, "number_of_particles"=w393, "min_FFT_power_value"=w392, "initial_pin_node"=w391, "accelerometer_mass"=w390) -> (w408:T13)  [unwired: 1 in]
      n184 = Build Path(base path=w439, name or relative path=w412) -> (appended path=w438:path)
      n185 = Flatten To JSON(anything=w408) -> (JSON string=w441:string)  [unwired: 2 in, 1 out]
      n186 = Write to Text File(file (use dialog)=w438, text=w441) -> (refnum out=w443:refnum<file>, error out=w442:errorcluster)  [unwired: 2 in, 1 out]
      n187 = Close File(refnum=w443, error in=w442) -> ()  [unwired: 2 out]
    }
  }
